vi "Write General Setting to File.vi"(11 "General Setup":T1={"Export Path"=path "C:/Glass", "level"=0.8, "Time Gap"=20.0}) -> ()   [LabVIEW 2015, in "ConfigHelper.lvlib"]
uses:
  ConfigHelper.lvlib
  Control_General Setup (Path).ctl
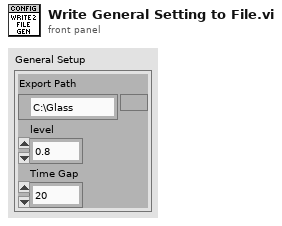
[diagram p1: front panel]
types:
  T1 = typedef "ConfigHelper.lvlib/Control_General Setup (Path).ctl" = cluster{"Export Path":path, "level":dbl, "Time Gap":dbl}
  T2 = typedef "ConfigHelper.lvlib/Control_General Setup (String).ctl" = cluster{"Export Path":string, "level":dbl, "Time Gap":dbl}
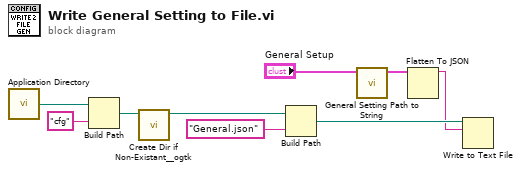
[diagram p0: block diagram]
diagram:
  n1 = call <vilib>:"Application Directory.vi"() -> ("Application Directory"=w9:path)
  n2 = Build Path(base path=w9, name or relative path="cfg") -> (appended path=w7:path)
  n3 = call <userlib>:"Create Dir if Non-Existant__ogtk.vi"("Directory Path"=w7) -> ("dup Directory Path"=w6:path)  [unwired: 8 in, 2 out]
  n4 = Build Path(base path=w6, name or relative path="General.json") -> (appended path=w4:path)
  n5 = call "General Setting Path to String.vi"("General Setup (Path)"="General Setup") -> ("General Setup (String)"=w1:T2)  [unwired: 10 in]
  n6 = Flatten To JSON(anything=w1) -> (JSON string=w3:string)  [unwired: 2 in, 1 out]
  n7 = Write to Text File(file (use dialog)=w4, text=w3) -> ()  [unwired: 2 in, 3 out]
